vi "CreateCaptionText.vi"(7 "Side":string="A - ", 8 "Serial":i32, 10 "ScannerReadOut":string[](array[string]), 11 "LaserVariables":string[](array[string])) -> (3 "Caption":string)   [LabVIEW 2016]
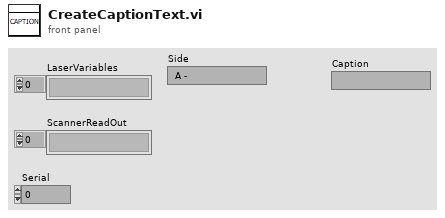
[diagram p1: front panel]
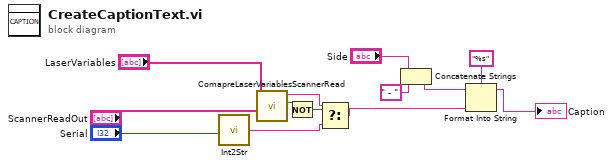
[diagram p0: block diagram]
diagram:
  n1 = call "Int2Str.vi"("Numeric"="Serial") -> ("string"=w11:string)
  n2 = call "ComapreLaserVariablesScannerRead.vi"("ScanerReadOut"="ScannerReadOut", "LaserVariables"="LaserVariables") -> ("Equals?"=w8:bool, "String"=w12:string)  [unwired: 8 in]
  n3 = Not(x=w8) -> (.not. x?=w10:bool)
  n4 = Select(t=w12, s=w10, f=w11) -> (s? t:f=w13:string)
  n5 = Concatenate Strings("Side", " - ") -> (w1:string)
  n6 = Format Into String(format string="%s", initial string=w1, w13) -> (resulting string=→"Caption":string)  [unwired: 1 in, 1 out]
